vi "Perform Auto Return.vi"(8 "error in (no error)":errorcluster, 10 "Auto Return?":bool, 11 "ESM303 in":refnum<class "ESM303.lvclass">) -> (0 "error out":errorcluster, 3 "ESM303 out":refnum<class "ESM303.lvclass">)   [LabVIEW 2018, in "ESM303.lvlib" / "ESM303.lvclass"]
uses:
  ESM303.lvclass
  builds/Force Test Stand/Force Test Stand/Force Test Stand.lvlibp/Force Test Stand.lvclass
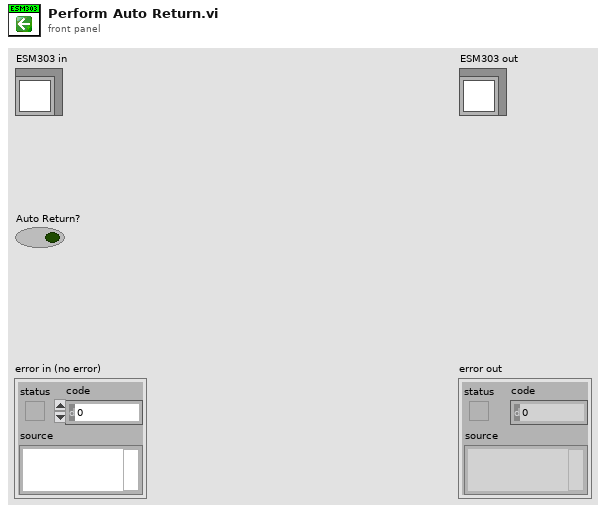
[diagram p1: front panel]
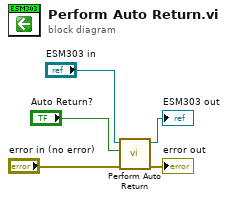
[diagram p0: block diagram]
diagram:
  n1 = call-parent "Perform Auto Return.vi"("error in (no error)"="error in (no error)", "Auto Return?"="Auto Return?", "Force Test Stand in"="ESM303 in") -> ("error out"=→"error out":errorcluster, "Force Test Stand out"=→"ESM303 out":refnum<class "ESM303.lvclass">)  [unwired: 7 in]
